vi "Test2.vi"() -> ()   [LabVIEW 2010]
panel:
  in  "Stop":bool
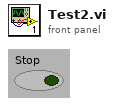
[diagram p1: front panel]
types:
  T1 = enum16{"Device 1", "Device 2", "Device 3", "Device 4", "Device 5", "Device 6", "Device 7", "Device 8"}
  T2 = enum8{"Input 1 (I1)", "Input 2 (I2)", "Input 3 (I3)", "Input 4 (I4)", "Input 5 (I5)", "Input 6 (I6)", "Input 7 (I7)", "Input 8 (I8)"}
  T3 = enum8{"Robo Interface", "Extension 1", "Extension 2", "Extension 3"}
  T4 = enum8{"Power 1", "Power 2", "Power 3", "Power 4", "Power 5", "Power 6", "Power 7", "Power 8"}
  T5 = enum8{"Output 1 (O1)", "Output 2 (O2)", "Output 3 (O3)", "Output 4 (O4)", "Output 5 (O5)", "Output 6 (O6)", "Output 7 (O7)", "Output 8 (O8)"}
  T6 = enum8{"Goes High", "Goes Low", "Goes High or Low"}
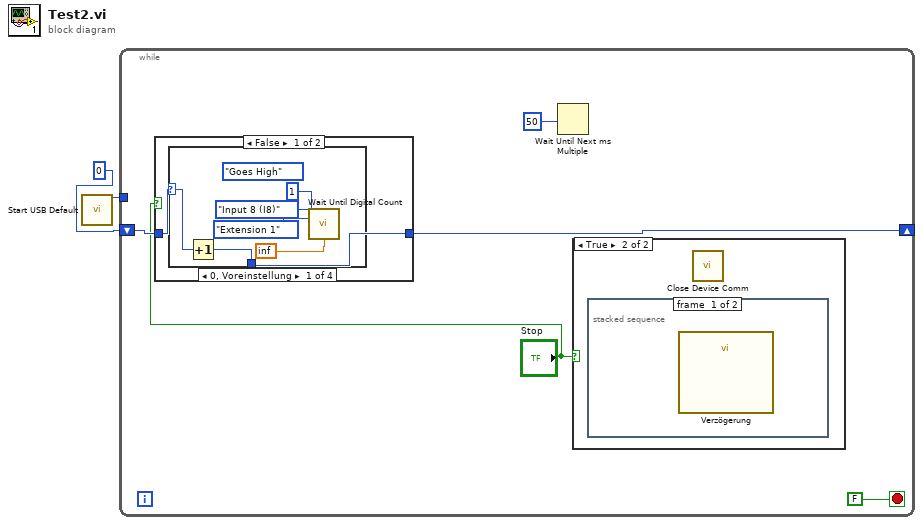
[diagram p0: block diagram]
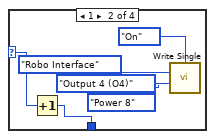
[diagram p2: hidden frame]
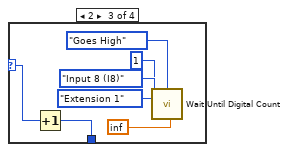
[diagram p3: hidden frame]
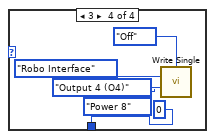
[diagram p4: hidden frame]
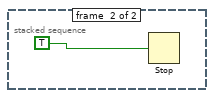
[diagram p7: hidden frame]
diagram:
  n1 = call "Start USB Default.vi"() -> ("Device ID Out"=w2:T1)  [unwired: 3 in, 12 out]
  n2 = while {
    tunnel: w2 -> [_]
    shift-right: [w4] -> _
    shift-left: 0 -> [w5]
    stop <- FALSE stop-if-true
    n3 = case shown="False" "Stop" {
      tunnel: w5 -> [w9 w34]
      tunnel: [w8 w34] -> w4
      frame False {
        n4 = case shown="0, Voreinstellung" w9 {
          selector: w9 -> [w11 w16 w22 _]
          tunnel: [w10 w17 w23 0] -> w8
          frame 0, Default {
            (unwired) T6."Goes High" ("Wait Until")
            n5 = Increment(x=w11) -> (x+1=w10:i32)
            n6 = call "Wait Until Digital Count.vi"("Module"=T3."Extension 1", "Digital_Input"=T2."Input 8 (I8)", "Final Count"=u32 1, "Time Out (10)"=inf) -> ()  [unwired: 3 in, 9 out]
          }
          frame 1 {
            n7 = Increment(x=w16) -> (x+1=w17:i32)
            n8 = call "Write Single.vi"("Output_Action"=enum8{"Off", "On"}."On", "Module"=T3."Robo Interface", "Single_Output"=T5."Output 4 (O4)", "Output_PWM"=T4."Power 8") -> ()  [unwired: 2 in, 10 out]
          }
          frame 2 {
            n9 = Increment(x=w22) -> (x+1=w23:i32)
            n10 = call "Wait Until Digital Count.vi"("Wait Until"=T6."Goes High", "Module"=T3."Extension 1", "Digital_Input"=T2."Input 8 (I8)", "Final Count"=u32 1, "Time Out (10)"=inf) -> ()  [unwired: 2 in, 9 out]
          }
          frame 3 {
            n11 = call "Write Single.vi"("Output_Action"=enum8{"Off", "On"}."Off", "Module"=T3."Robo Interface", "Single_Output"=T5."Output 4 (O4)", "Output_PWM"=T4."Power 8") -> ()  [unwired: 2 in, 10 out]
          }
        }
      }
      frame True {
      }
    }
    n12 = Wait Until Next ms Multiple(millisecond multiple=50) -> ()  [unwired: 1 out]
    n13 = case shown="True" "Stop" {
      frame False {
      }
      frame True {
        n14 = stacked-sequence {
          frame #0 {
            n15 = call "Verzögerung"() -> ()  [unwired: 2 in, 10 out]
          }
          frame #1 {
            n16 = Stop(stop? (T)=TRUE) -> ()
          }
        }
        n17 = call "Close Device Comm.vi"() -> ()  [unwired: 2 in, 14 out]
      }
    }
  }
